vi "Initialize.vi"(7 "writer buffer size":i32, 8 "error in (no error)":errorcluster, 9 "reader url":string, 10 "writer name":string) -> (0 "error out":errorcluster, 3 "NetworkStreamWriter out":refnum<class "NetworkStreamWriter.lvclass">)   [LabVIEW 2011, in "NetworkStreamWriter.lvclass"]
doc: "This VI returns an instance of the NetworkStreamWriter class. A NetworkStreamWriter attempts to open a network stream with a reader endpoint. As with network streams, the writer url on the reader or the reader url on the writer must be given before the connection can be made. Note that until a connection is made, this VI will not return. It will, however, stop on a commanded e-stop from the top-level VI. This VI also launches a writer daemon which constantly sends information added to the internal queue by the Write method across the network stream."
uses:
  NetworkStreamWriter.lvclass
  Shared/messageQueue.ctl
  Shared/message.ctl
  NetworkStreamWriter.lvclass/NetworkStreamWriter.ctl
  WriterDaemon.vi
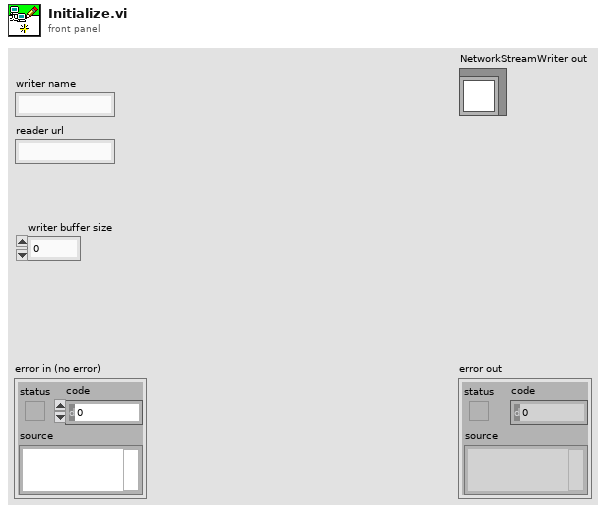
[diagram p1: front panel]
types:
  T1 = typedef "messageQueue.ctl" = refnum<queue>
  T2 = typedef "message.ctl" = cluster{"Data":variant, "Time since start (s)":dbl}
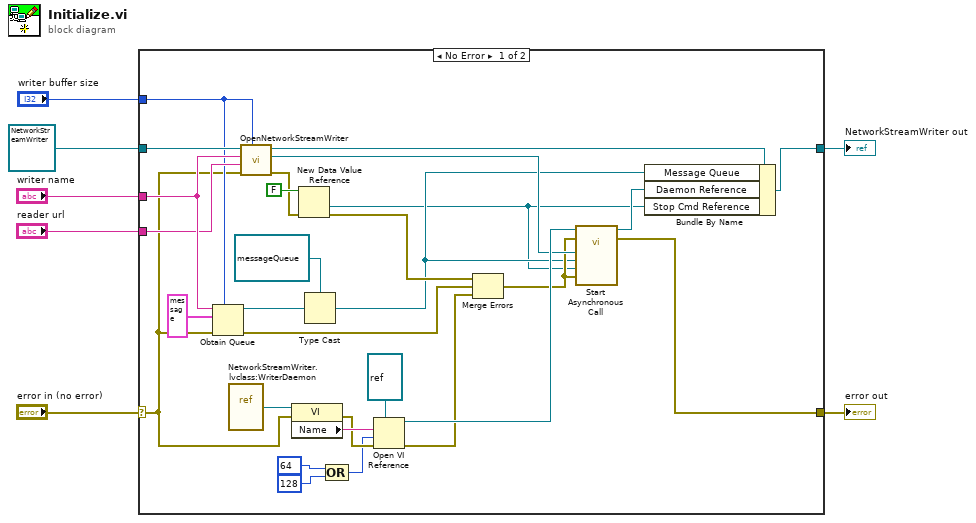
[diagram p0: block diagram]
diagram:
  n1 = case shown="No Error" "error in (no error)" {
    selector: "error in (no error)" -> [w26 w38]
    tunnel: [w21 w38] -> w6
    tunnel: [w31 w37] -> w5
    tunnel: refnum<class "NetworkStreamWriter.lvclass"> refnum ("NetworkStreamWriter in") -> [w36 w37]
    tunnel: "writer name" -> [w35 _]
    tunnel: "reader url" -> [w34 _]
    tunnel: "writer buffer size" -> [w32 _]
    frame No Error {
      n2 = Obtain Queue(max queue size (-1, unlimited)=w32, name (unnamed)=w35, element data type=T2 {"Data"=variant, "Time since start (s)"=0.0}, error in (no error)=w26) -> (queue out=w12:refnum<queue>, error out=w23:errorcluster)  [unwired: 1 in, 1 out]
      n3 = vi-ref "NetworkStreamWriter.lvclass:WriterDaemon.vi"() -> (w30:refnum<vi>)
      n4 = call "OpenNetworkStreamWriter.vi"("writer buffer size"=w32, "error in (no error)"=w26, "reader url"=w34, "writer name"=w35, "NetworkStreamWriter in"=w36) -> ("error out"=w14:errorcluster, "Writer Endpoint"=w22:refnum<k21>, "NetworkStreamWriter out"=w8:refnum<class "NetworkStreamWriter.lvclass">)  [unwired: 4 in]
      n5 = property class="VI"(reference=w30, error in=w26) -> (error out=w25:errorcluster, "Name"=w29:string)  [unwired: 1 out]
      n6 = New Data Value Reference(data value=FALSE, error in=w14) -> (data value reference=w9:refnum<data-value>, error out=w13:errorcluster)
      n7 = Type Cast(type=T1 refnum ("Variant Queue"), x=w12) -> (*(type *) &x=w10:T1)
      n8 = Compound Arithmetic op=OR(64 ("options"), 128 ("options")) -> (w16:i32)
      n9 = Open VI Reference(type specifier VI Refnum (for type only)=refnum<vi> refnum, vi path=w29, options=w16, error in (no error)=w25) -> (vi reference=w28:refnum<vi>, error out=w24:errorcluster)  [unwired: 2 in]
      n10 = Merge Errors(w13, w23, w24) -> (w20:errorcluster)
      n11 = call-by-ref "Start Asynchronous Call"(reference=w28, error in=w20, 8:"error in (no error)"=w20, "Stop Cmd Reference"=w9, "Message Queue"=w10, "Writer Endpoint"=w22) -> (reference out=w19:refnum<vi>, error out=w21:errorcluster)  [unwired: 8 in]
      n12 = Bundle By Name(cluster=w8, "Message Queue"=w10, "Daemon Reference"=w19, "Stop Cmd Reference"=w9) -> (w31:refnum<class "NetworkStreamWriter.lvclass">)
    }
    frame Error {
    }
  }
  "error out" <- w6
  "NetworkStreamWriter out" <- w5
